vi "zmq_get_monitor.vi"(6 "error in":errorcluster, 9 "monitor in":refnum<class "Socket.lvclass">) -> (0 "error out":errorcluster, 2 "event":T1, 3 "monitor out":refnum<class "Socket.lvclass">, 4 "addr":string, 5 "value":i32)   [LabVIEW 2025]
doc: "Receive a montor message from the provided socket and decodes it into readable form. The type of the event, associated endpoint address, and event-specific integer are returned.\n\nThis is a blocking call, and will terminate with the monitor socket.\n\nDetails on the event data: http://api.zeromq.org/3-2:zmq-socket-monitor"
uses:
  Socket.lvclass/Socket.ctl
  Socket.lvclass
  ZeroMQ.lvlib
  monitor_event.ctl
panel:
  # "ØMQ"
  # "labview"
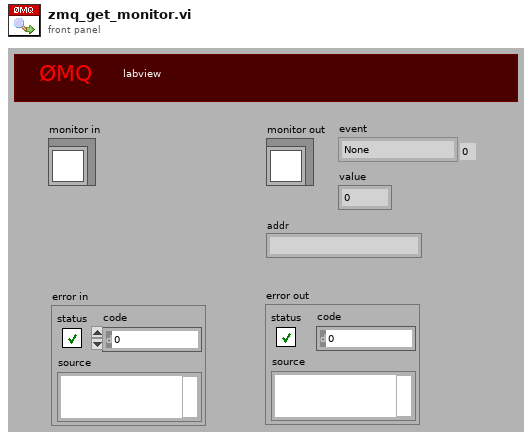
[diagram p1: front panel]
types:
  T1 = typedef "ZeroMQ.lvlib/monitor_event.ctl" = enum8{"None", "Connected", "Connect Delayed", "Connect Retry", "Listening", "Bind Failed", "Accepted", "Accept Failed", "Closed", "Close Failed", "Disconnected", "Monitor Stopped"}
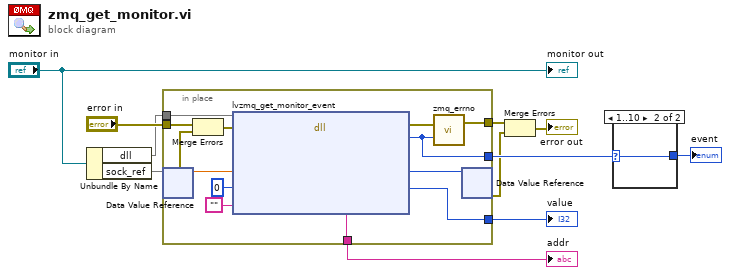
[diagram p0: block diagram]
diagram:
  n1 = Unbundle By Name("monitor in") -> ("dll"=w1, "sock_ref"=w9)
  n2 = in-place {
    in-place-border: "error in" -> [w23]
    in-place-border: [w22] -> w4
    in-place-border: [w21] -> w7
    in-place-border: [w16] -> w6
    in-place-border: [w15] -> w8
    in-place-border: w1 -> [w12]
    n3 = in-place-dvr #1(w9) -> (w20:dbl, w13:errorcluster)
    n4 = Merge Errors(w23, w13) -> (w14:errorcluster)
    n5 = dll-call lib="?" fn="lvzmq_get_monitor_event" ("zmq_labview.dll:lvzmq_socket")(path in=w12, error in=w14, "sock_obj"=w20, "intval"=0, "addr"="") -> (error out=w24:errorcluster, "return type"=w16:i32, "sock_obj"=w19:u64, "intval"=w15:i32, "addr"=w21:string)  [unwired: 3 in, 1 out]
    n6 = call "zmq_errno.vi"("retval"=w16, "error in"=w24) -> ("error out"=w22:errorcluster)  [unwired: 1 out]
    n7 = in-place-dvr #1(w19) -> (w3:errorcluster)  [unwired: 1 out]
  }
  "addr" <- w7
  "value" <- w8
  n8 = Merge Errors(w4, w3) -> (→"error out":errorcluster)
  n9 = case shown="1..10" w6 {
    selector: w6 -> [_ w25]
    tunnel: [_ w25] -> w5
    frame Default {
    }
    frame 1..10 {
    }
  }
  "event" <- w5
  "monitor out" <- "monitor in"
